vi "FiberWLCLwrapExtract.vi"(7 "median filter (points)":i32=5, 9 "params in (all)":dbl[](array[numeric])=[0.0, 0.0, 6000.0, 50.0, 900.0, 197.0, 1.7, 0.3, 105.0, 80.0, 17.0, 5.0], 10 "tracename":string="E:\\users\\noort\\data\\270404\\_001.log", 11 "Stepsize (bp)":i32=5) -> (1 "Channel data":dbl[][](array[numeric]), 2 "Channels":string[](array[string]), 3 "Lwrap (bp)":i16[](graph))   [LabVIEW 2018]
uses:
  <vilib>/Analysis/1siggen.llb/Ramp Pattern by Delta.vi
  <vilib>/Analysis/NI_AALBase.lvlib
  <vilib>/Analysis/NI_AAL_SigProc.lvlib
  <vilib>/gmath/NI_Gmath.lvlib
panel:
  out "XY Graph 2":cluster{"Data out":dbl[], dbl[]}(graph)
  out "XY Graph":cluster{"Data out":dbl[], "Data out":dbl[]}[](graph)
  out "# found":i32
  out "Pwrap(Lwrap)":T1(graph)
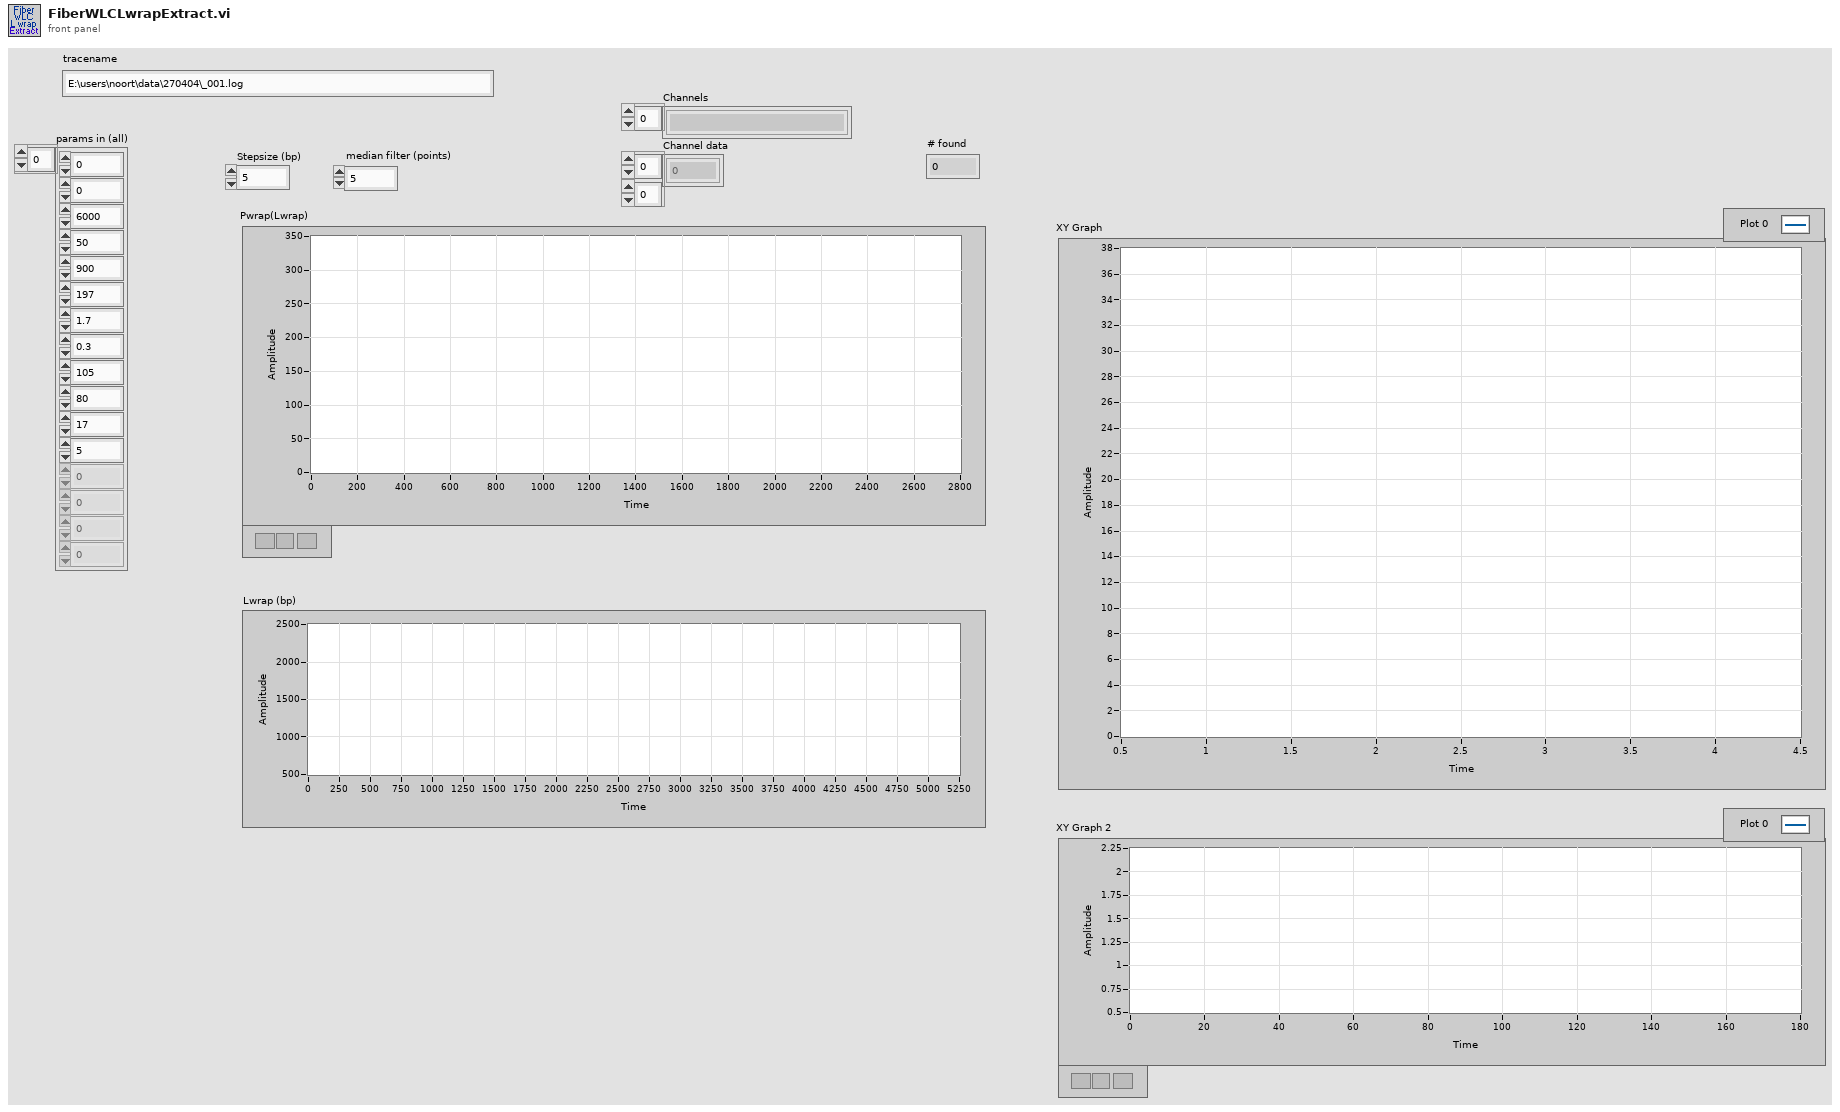
[diagram p1: front panel]
types:
  T1 = cluster{"Ramp Pattern":dbl[], "Amplitudes":dbl[]}[]
  T2 = enum16{"Read", "Write", "Get channels", "Delete channels"}
  T3 = enum16{"Z0 (nm)", "dZ/dt (nm/s)", "L (bp)", "P (nm)", "S (pN)", "NRL (bp)", "NLD (nm)", "k (pN/nm)", "Lwrap1 (bp)", "Lwrap2 (bp)", "N4+N8", "N4"}
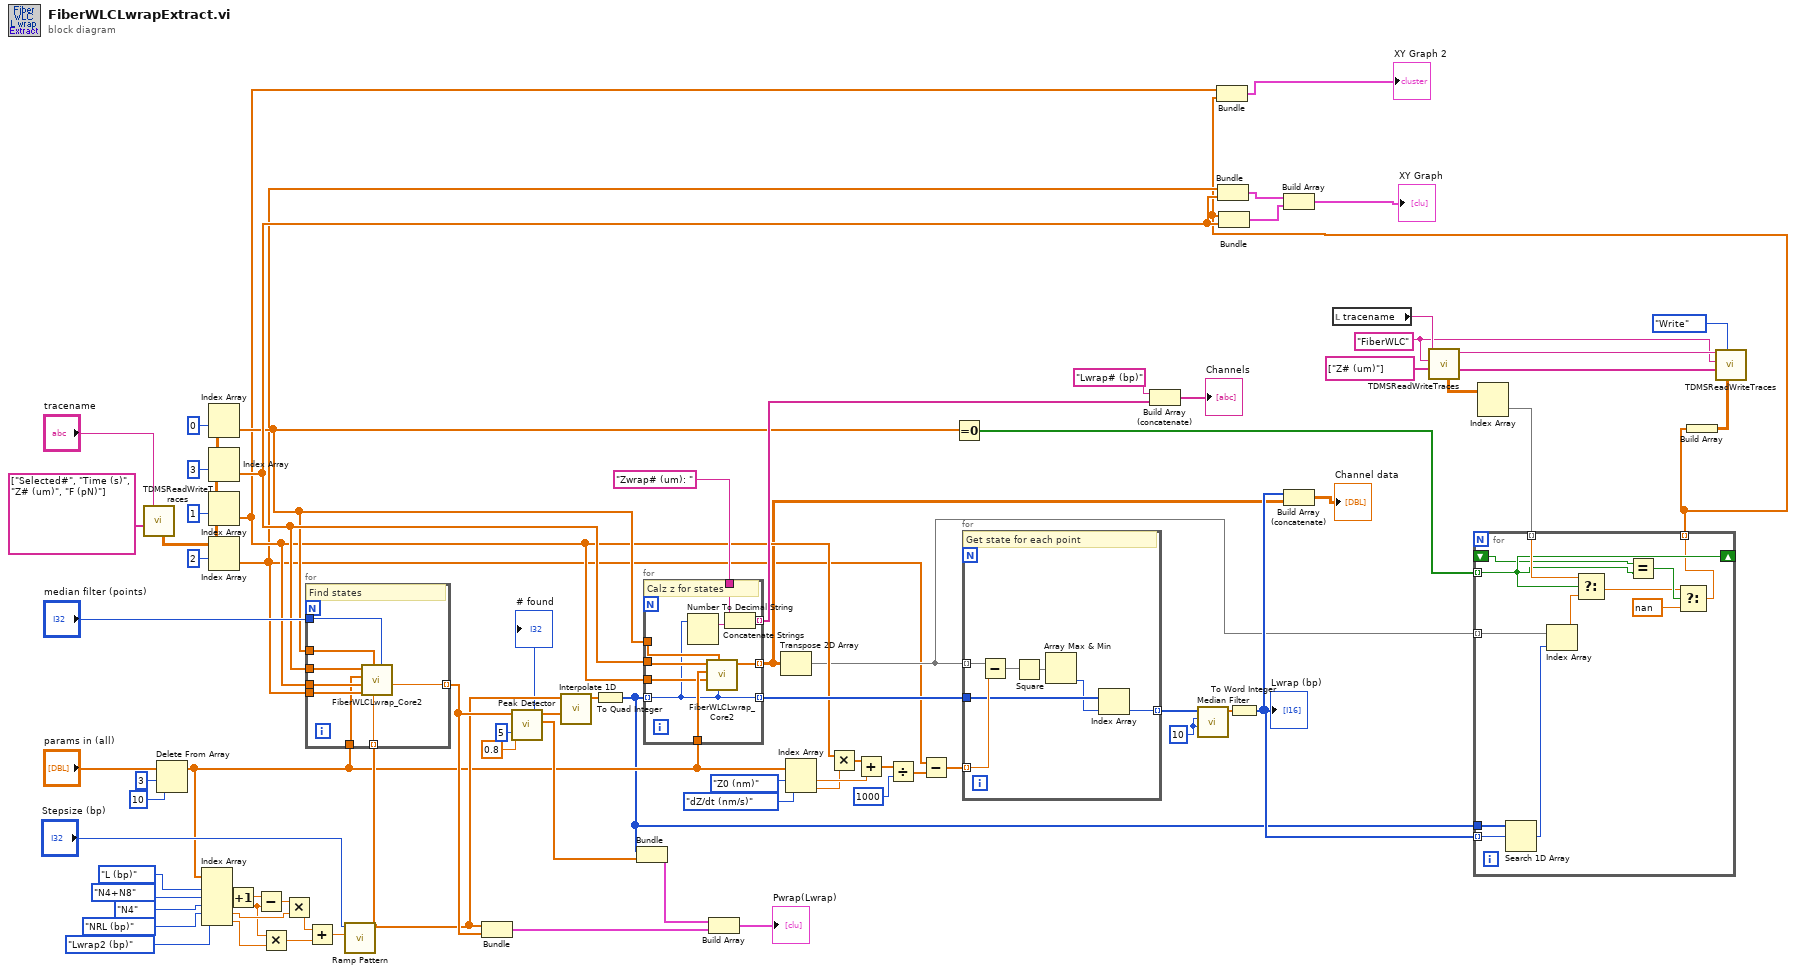
[diagram p0: block diagram]
diagram:
  w3 = "FiberWLC" ("group name")
  w53 = 10 ("left rank")
  n1 = call "TDMSReadWriteTraces.vi"("Channels in"=string[] ["Selected#", "Time (s)", "Z# (um)", "F (pN)"] ("channel name(s) in"), "tracename"="tracename") -> ("Data out"=w44:dbl[][])  [unwired: 4 in, 5 out]
  n2 = Delete From Array(array="params in (all)", length=3, index=10) -> (array with subset deleted=w33:dbl[])  [unwired: 1 out]
  n3 = Index Array(array=w33, index #1=T3."L (bp)" ("Pars (Do not change)"), index #2=T3."N4+N8" ("Pars (Do not change)"), index #3=T3."N4" ("Pars (Do not change)"), index #4=T3."NRL (bp)" ("Pars (Do not change)"), index #5=T3."Lwrap2 (bp)" ("Pars (Do not change)")) -> (element #2=w70:dbl, element #3=w66:dbl, element #4=w69:dbl, element #5=w65:dbl)  [unwired: 1 out]
  n4 = Index Array(array=w44, index (row)=0) -> (element=w21:dbl[])  [unwired: 1 in]
  n5 = Index Array(array=w44, index (row)=3) -> (element=w26:dbl[])  [unwired: 1 in]
  n6 = Index Array(array=w44, index (row)=1) -> (element=w19:dbl[])  [unwired: 1 in]
  n7 = Index Array(array=w44, index (row)=2) -> (element=w12:dbl[])  [unwired: 1 in]
  n8 = Increment(x=w70) -> (x+1=w1:dbl)
  n9 = Subtract(x=w1, y=w66) -> (x-y=w67:dbl)
  n10 = Multiply(x=w66, y=w65) -> (x*y=w64:dbl)
  n11 = Multiply(x=w67, y=w69) -> (x*y=w63:dbl)
  n12 = Add(x=w63, y=w64) -> (x+y=w39:dbl)
  n13 = call-poly <vilib>:"Ramp Pattern.vi"("end"=w39, "delta"="Stepsize (bp)") -> ("Ramp Pattern"=w74:dbl[])  [unwired: 7 in, 2 out]
  n14 = for {
    tunnel: w26 -> [w87]
    tunnel: w19 -> [w86]
    tunnel: w12 -> [w85]
    tunnel: w33 -> [w84]
    tunnel: w21 -> [w83]
    tunnel: w74 -> [w82] mode=indexing
    tunnel: [w81] -> w75 mode=indexing
    tunnel: "median filter (points)" -> [w80]
    # "Find states"
    n15 = call "FiberWLCLwrap_Core2.vi"("median filter (points)"=w80, "Lwrap"=w82, "selected (0,1)"=w83, "z in (um)"=w85, "t (s)"=w86, "params in (all)"=w84, "F (pN)"=w87) -> ("SumP(Lwrap)"=w81:dbl)  [unwired: 1 in, 3 out]
  }
  n16 = Bundle("Ramp Pattern"=w74, w75) -> (w48:cluster{"Ramp Pattern":dbl[], dbl[]})  [unwired: 1 in]
  n17 = call <vilib>:"Peak Detector.vi"("width"=5, "threshold"=0.8, "X"=w75) -> ("Amplitudes"=w50:dbl[], "Locations"=w76:dbl[], "# found"=→"# found":i32)  [unwired: 4 in, 2 out]
  n18 = call <vilib>:"Interpolate 1D.vi"("xi"=w76, "Y"=w74) -> ("yi"=w14:dbl[])  [unwired: 7 in, 2 out]
  n19 = To Quad Integer(1:w14) -> (0:w13:i64[])
  n20 = Bundle(w13, "Amplitudes"=w50) -> (w49:cluster{i64[], "Amplitudes":dbl[]})  [unwired: 1 in]
  n21 = for {
    tunnel: w33 -> [w96]
    tunnel: w21 -> [w95]
    tunnel: w26 -> [w94]
    tunnel: w19 -> [w93]
    tunnel: [w92] -> w17 mode=indexing
    tunnel: w13 -> [w88] mode=indexing
    tunnel: [w88] -> w55 mode=indexing
    tunnel: "Zwrap# (um): " -> [w90]
    tunnel: [w89] -> w30 mode=indexing
    # "Calz z for states"
    n22 = Number To Decimal String(number=w88) -> (decimal integer string=w91:string)  [unwired: 1 in]
    n23 = call "FiberWLCLwrap_Core2.vi"("Lwrap"=w88, "selected (0,1)"=w95, "t (s)"=w93, "params in (all)"=w96, "F (pN)"=w94) -> ("z out (um)"=w92:dbl[])  [unwired: 3 in, 3 out]
    n24 = Concatenate Strings(w90, w91) -> (w89:string)
  }
  n25 = Build Array(w49, w48) -> (→"Pwrap(Lwrap)":T1)
  n26 = Transpose 2D Array(2D array=w17) -> (transposed array=w16:dbl[][])
  n27 = Index Array(array=w33, index #1=T3."Z0 (nm)" ("Pars (Do not change)"), index #2=T3."dZ/dt (nm/s)" ("Pars (Do not change)")) -> (element #1=w62:dbl, element #2=w60:dbl)
  n28 = Multiply(x=w19, y=w60) -> (x*y=w61:dbl[])
  n29 = Add(x=w61, y=w62) -> (x+y=w37:dbl[])
  n30 = Divide(x=w37, y=1000 ("width")) -> (x/y=w56:dbl[])
  n31 = Subtract(x=w12, y=w56) -> (x-y=w38:dbl[])
  n32 = Equal To 0?(x=w21) -> (x = 0?=w15:bool[])
  n33 = for {
    tunnel: w16 -> [w98] mode=indexing
    tunnel: w38 -> [w103] mode=indexing
    tunnel: w55 -> [w102]
    tunnel: [w99] -> w54 mode=indexing
    # "Get state for each point"
    n34 = Subtract(x=w98, y=w103) -> (x-y=w101:dbl[])
    n35 = Square(x=w101) -> (x^2=w100:dbl[])
    n36 = Array Max & Min(array=w100) -> (min index (indices)=w97:i32)  [unwired: 3 out]
    n37 = Index Array(array=w102, index=w97) -> (element=w99:i64)
  }
  n38 = Build Array (concatenate)("Lwrap# (bp)", w30) -> (→"Channels":string[])
  n39 = call <vilib>:"Median Filter.vi"("right rank"=w53, "left rank"=w53, "X"=w54) -> ("Filtered X"=w52:dbl[])  [unwired: 7 in, 1 out]
  n40 = Bundle("Data out"=w12, "Data out"=w26) -> (w25:cluster{"Data out":dbl[], "Data out":dbl[]})  [unwired: 1 in]
  n41 = To Word Integer(number=w52) -> (16bit integer=w20:i16[])
  "Lwrap (bp)" <- w20
  n42 = Build Array (concatenate)(w20, w17) -> (→"Channel data":dbl[][])
  n43 = local read "tracename"() -> (w11:string)
  n44 = call "TDMSReadWriteTraces.vi"("Channels in"=string[] ["Z# (um)"], "group name"=w3, "tracename"=w11) -> ("Channels out"=w7:string[], "tracename out"=w8:string, "Data out"=w10:dbl[][])  [unwired: 3 in, 3 out]
  n45 = Index Array(array=w10) -> (element=w9:dbl[])  [unwired: 2 in]
  n46 = for {
    tunnel: w20 -> [w114] mode=indexing
    tunnel: w13 -> [w115]
    tunnel: w16 -> [w113] mode=indexing
    tunnel: [w104] -> w6 mode=indexing
    tunnel: w15 -> [w109] mode=indexing
    tunnel: w9 -> [w110] mode=indexing
    shift-right: [w109] -> _
    shift-left: _ -> [w108]
    n47 = Search 1D Array(1D array=w115, element=w114) -> (index of element=w112:i32)  [unwired: 1 in]
    n48 = Index Array(array=w113, index=w112) -> (element=w111:dbl)
    n49 = Select(t=w110, s=w109, f=w111) -> (s? t:f=w106:dbl)
    n50 = Equal?(x=w108, y=w109) -> (x = y?=w107:bool)
    n51 = Select(t=w106, s=w107, f=nan) -> (s? t:f=w104:dbl)
  }
  n52 = Bundle("Data out"=w19, w6) -> (→"XY Graph 2":cluster{"Data out":dbl[], dbl[]})  [unwired: 1 in]
  n53 = Bundle(w6, "Data out"=w26) -> (w24:cluster{dbl[], "Data out":dbl[]})  [unwired: 1 in]
  n54 = Build Array(w25, w24) -> (→"XY Graph":cluster{"Data out":dbl[], "Data out":dbl[]}[])
  n55 = Build Array(w6) -> (w5:dbl[][])
  n56 = call "TDMSReadWriteTraces.vi"("Data in"=w5, "Task"=T2."Write", "Channels in"=w7, "group name"=w3, "tracename"=w8) -> ()  [unwired: 1 in, 6 out]
